vi "Clase2.vi"() -> ()   [LabVIEW 2011]
panel:
  out "Temperatura agradable":bool
  out "Alarma":bool
  out "ValorTemperatura":dbl
  out "Temperatura":i32(slide) scale=0.0..60.0
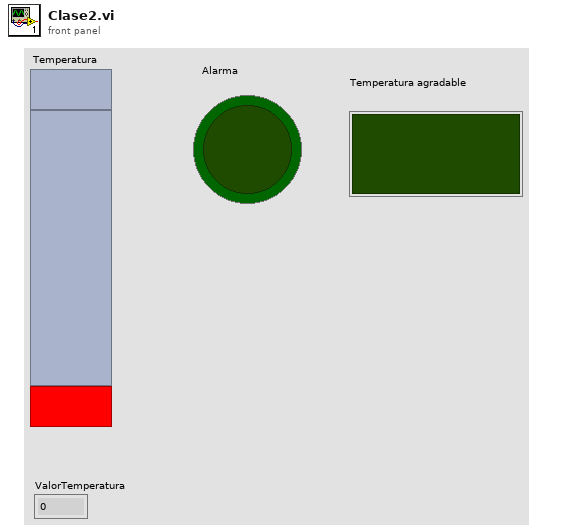
[diagram p1: front panel]
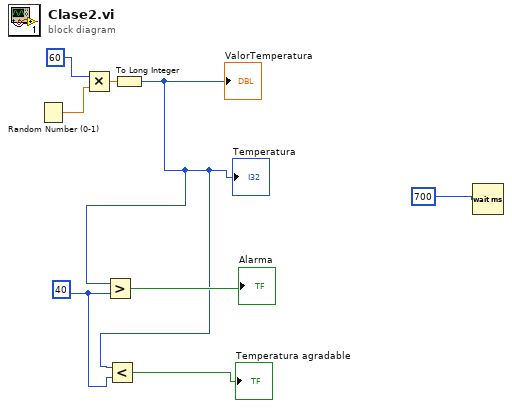
[diagram p0: block diagram]
diagram:
  w3 = 40
  n1 = Random Number (0-1)() -> (number: 0 to 1=w7:dbl)
  n2 = Multiply(x=60, y=w7) -> (x*y=w6:dbl)
  n3 = To Long Integer(number=w6) -> (32bit integer=w2:i32)
  "Temperatura" <- w2
  "ValorTemperatura" <- w2
  n4 = Greater?(x=w2, y=w3) -> (0:→"Alarma":bool)
  n5 = Less?(x=w2, y=w3) -> (x < y?=→"Temperatura agradable":bool)
  n6 = Wait (ms)(milliseconds to wait=700) -> ()  [unwired: 1 out]
